vi "Test 3.vi"(8 "error in (no error)":errorcluster, 11 "Test Case In":refnum<class "Tests.lvclass">) -> (0 "error out":errorcluster, 3 "Test Case Out":refnum<class "Tests.lvclass">)   [LabVIEW 2020, in "Tests.lvclass"]
uses:
  Tests.lvclass
  C:/Program Files (x86)/National Instruments/LabVIEW 2020/vi.lib/Astemes/LUnit/Test Case.lvclass
  <vilib>/Astemes/LUnit/Test Case.lvclass/Test Case.ctl
  <vilib>/Astemes/LUnit/Append Fail Result.vi
  <vilib>/Astemes/LUnit/Append Pass Result.vi
  <vilib>/Astemes/LUnit/Run In UI.vi
  <vilib>/Utility/error.llb/Clear Errors.vi
  Tests.lvclass/Tests.ctl
  Proto/Proto.lvclass
  <vilib>/Astemes/LUnit/Test Case.lvclass
  C:/Program Files (x86)/National Instruments/LabVIEW 2020/vi.lib/Astemes/LUnit/LUnit Runnable.lvclass
  C:/git/aoc-2023/Day 24_24/Tests/Tests.lvclass
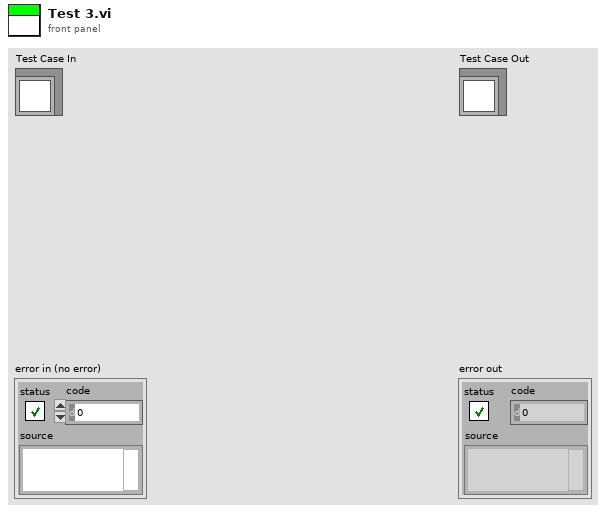
[diagram p1: front panel]
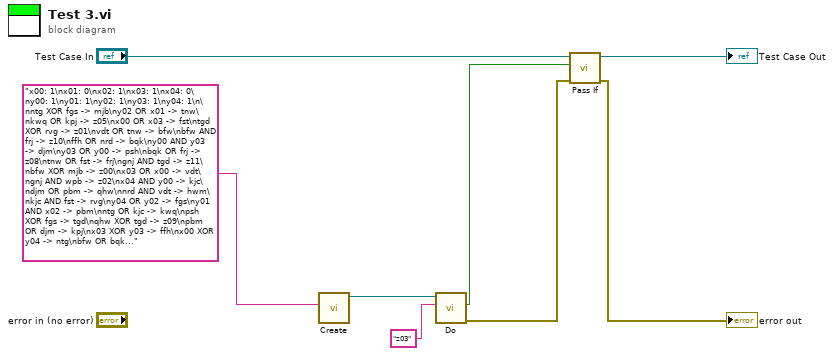
[diagram p0: block diagram]
diagram:
  n1 = call "Create.vi"("Input"="x00: 1\nx01: 0\nx02: 1\nx03: 1\nx04: 0\ny00: 1\ny01: 1\ny02: 1\ny03: 1\ny04: 1\n\nntg XOR fgs -> mjb\ny02 OR x01 -> tnw\nkwq OR kpj -> z05\nx00 OR x03 -> fst\ntgd XOR rvg -> z01\nvdt OR tnw -> bfw\nbfw AND frj -> z10\nffh OR nrd -> bqk\ny00 AND y03 -> djm\ny03 OR y00 -> psh\nbqk OR frj -> z08\ntnw OR fst -> frj\ngnj AND tgd -> z11\nbfw XOR mjb -> z00\nx03 OR x00 -> vdt\ngnj AND wpb -> z02\nx04 AND y00 -> kjc\ndjm OR pbm -> qhw\nnrd AND vdt -> hwm\nkjc AND fst -> rvg\ny04 OR y02 -> fgs\ny01 AND x02 -> pbm\nntg OR kjc -> kwq\npsh XOR fgs -> tgd\nqhw XOR tgd -> z09\npbm OR djm -> kpj\nx03 XOR y03 -> ffh\nx00 XOR y04 -> ntg\nbfw OR bqk -> z06\nnrd XOR fgs -> wpb\nfrj XOR qhw -> z04\nbqk OR frj -> z07\ny03 OR x01 -> nrd\nhwm AND bqk -> z03\ntgd XOR rvg -> z12\ntnw OR pbm -> gnj") -> ("Proto"=w4:refnum<class "Proto.lvclass">)  [unwired: 10 in]
  n2 = call "Do.vi"("Key"="z03", "Proto in"=w4) -> ("error out"=w5:errorcluster, "Value"=w1:bool)  [unwired: 7 in, 1 out]
  n3 = call <vilib>:"Pass If.vi"("error in (no error)"=w5, "Pass?"=w1, "LUnit Test Case In"="Test Case In") -> ("error out"=→"error out":errorcluster, "LUnit Test Case Out"=→"Test Case Out":refnum<class "Tests.lvclass">)  [unwired: 7 in]
